vi "controlEffort.vi"(7 "Inverted?":bool, 10 "Enable":bool, 11 "force":dbl) -> ()   [LabVIEW 2013]
uses:
  <vilib>/myRIO/Instrument Drivers/Onboard IO/PWM/vis/Smart Open.vi
  <vilib>/myRIO/Instrument Drivers/Onboard IO/PWM/vis/Set Duty Cycle and Frequency.vi
  <vilib>/myRIO/Instrument Drivers/Onboard IO/DIO/vis/Smart Open.vi
  <vilib>/myRIO/Instrument Drivers/Onboard IO/DIO/vis/Write.vi
  <vilib>/myRIO/Instrument Drivers/Onboard IO/PWM/vis/Open.vi
  <vilib>/myRIO/Instrument Drivers/Onboard IO/DIO/vis/Open.vi
  <vilib>/imath/engines/lvmath2/RunTimeEngine/NodeEndStatement/NIMS_NodeEndStatement_Output.vi
  <instcachedir>/0/NIMS_NodeEndStatement_Output_53EC0D466D134D7ABD903AC30B43404B.lvgen/NIMS_NodeEndStatement_Output_53EC0D466D134D7ABD903AC30B43404B_001.vi
  <vilib>/imath/engines/lvmath2/RunTimeEngine/ErrorHandling/NIMS_Finalize Error.vi
  <vilib>/Utility/error.llb/Error Cluster From Error Code.vi
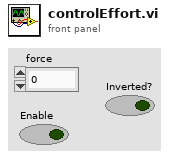
[diagram p1: front panel]
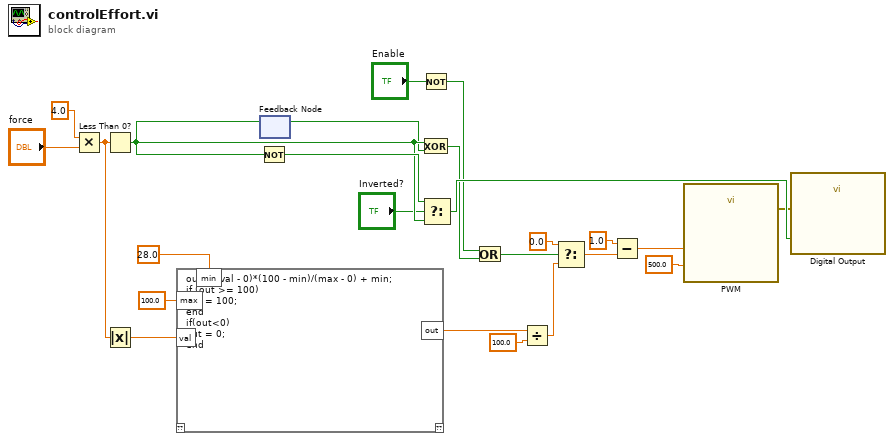
[diagram p0: block diagram]
diagram:
  n1 = Multiply(x=4.0, y="force") -> (x*y=w3:dbl)
  n2 = Less Than 0?(x=w3) -> (x < 0?=w23:bool)
  n3 = Absolute Value ("Absolute Value 2")(x=w3) -> (abs(x)=w17:dbl)
  n4 = mathscript code="out = (val - 0)*(100 - min)/(max - 0) + min;\nif (out >= 100)\nout = 100;\nend\nif(out<0)\nout = 0;\nend"("val"=w17, "max"=100.0 ("max_in"), "min"=28.0 ("min_out")) -> ("out"=w19:dbl)  [unwired: 1 in, 1 out]
  n5 = Not ("Not 2")(x=w23) -> (.not. x?=w24:bool)
  n6 = feedback #1 ("Feedback Node 2")() -> (w12:bool)  [unwired: 1 in]
  n7 = feedback-in #1 ("3")(w23) -> ()
  n8 = Not(x="Enable") -> (.not. x?=w9:bool)
  n9 = Exclusive Or(1:w12, 2:w23) -> (0:w8:bool)
  n10 = Select ("Select 2")(t=w24, s="Inverted?", f=w23) -> (s? t:f=w16:bool)
  n11 = Or ("Or 2")(x=w9, y=w8) -> (x .or. y?=w11:bool)
  n12 = Divide(x=w19, y=100.0 ("y 3")) -> (x/y=w21:dbl)
  n13 = Select(t=0.0, s=w11, f=w21) -> (s? t:f=w7:dbl)
  n14 = Subtract(x=1.0, y=w7) -> (x-y=w14:dbl)
  n15 = call "PWM"("Duty Cycle (0-1)"=w14, "Frequency (Hz)"=500.0 ("pwm freq")) -> ("error out"=w4:errorcluster)  [unwired: 25 in]
  n16 = call "Digital Output"("A/DIO6 (Pin 23)"=w16, "error in (no error)"=w4) -> ()  [unwired: 25 in, 1 out]
